vi "Main_v2.vi"() -> ()   [LabVIEW 2018]
uses:
  <vilib>/platform/TimedLoop/XDataNode/XDataNode.xnode
  <vilib>/Platform/TimedLoop/XDataNode/nitl_modes.ctl
  <vilib>/Platform/TimedLoop/XDataNode/XDNodeRunTimeDep.lvlib
  <vilib>/Platform/TimedLoop/XDataNode/wakeup.ctl
  <vilib>/Platform/TimedLoop/XDataNode/timing_clust.ctl
  Clusters/RoscoParams.ctl
  Clusters/SwapIn.ctl
  Clusters/SwapIndexes.ctl
  Clusters/FileDataChannel.ctl
  Clusters/SimulationConstants.ctl
panel:
  out "Generator Speed (rad/s)":sgl(slide)=7.06858e-05 scale=-4.0..4.0
  in  "?":T1(tab)
  out "Generator Speed":sgl(graph)
  out "Torque Setpoint (kNm)":sgl(graph)
  out "Pitch Setpoint":sgl(graph)
  in  "To VS_ControlMode":T2(ring)
  in  "Edit DISCON":bool
  out "DISCON.IN Contents":string
  in  "From VS_ControlMode":T2(ring)
  in  "GenSpeeed Amplitude":sgl=0.5
  in  "GenSpeed Mean":sgl=0.5
  out "Rotor Speed (rad/s)":sgl(slide)=7.06858e-05 scale=-4.0..4.0
  out "Torque Setpoint (kNm)":sgl(knob) scale=0.0..21586451.0
  out "Pitch Setpoint":sgl(knob) scale=0.0..1.5
  out "Power (kW)":sgl(slide) scale=-15000.0..15000.0 scale format="%.2f"
  in  "Init WindSpeed(m/s)":sgl=7.0
  in  "File path":path=path "/home/lvuser/rosco-tests"
  out "SimLoop Late?":bool
  out "FIFO Loop Late?":bool
  in  "Base filename":string="rosco-tests"
  out "Writing to cRIO?":bool
  in  "WriteData":bool
  in  "?":T3
  out "#RT FIFO":u32
  out "Call to Rosco Failed?":bool
  out "Rosco Return Message":string
  in  "?":bool
  out "time(s)":dbl
  out "RT Loop Late?":bool
  # "FOCAL Realtime Control (IEA 15MW)"
  # "SENSOR INPUTS"
  # "FILEWRITING SETTINGS"
  # "ERRORS"
  # "TURBINE SPECIFICATIONS"
  # "ROSCO OUTPUTS"
  # "RATED POWER: 15000000 W"
  # "RATED TORQUE: 19624046.66 Nm"
  # "RATED GEN SPEED: 0.79168 rad/s"
  # "ROSCO INPUTS"
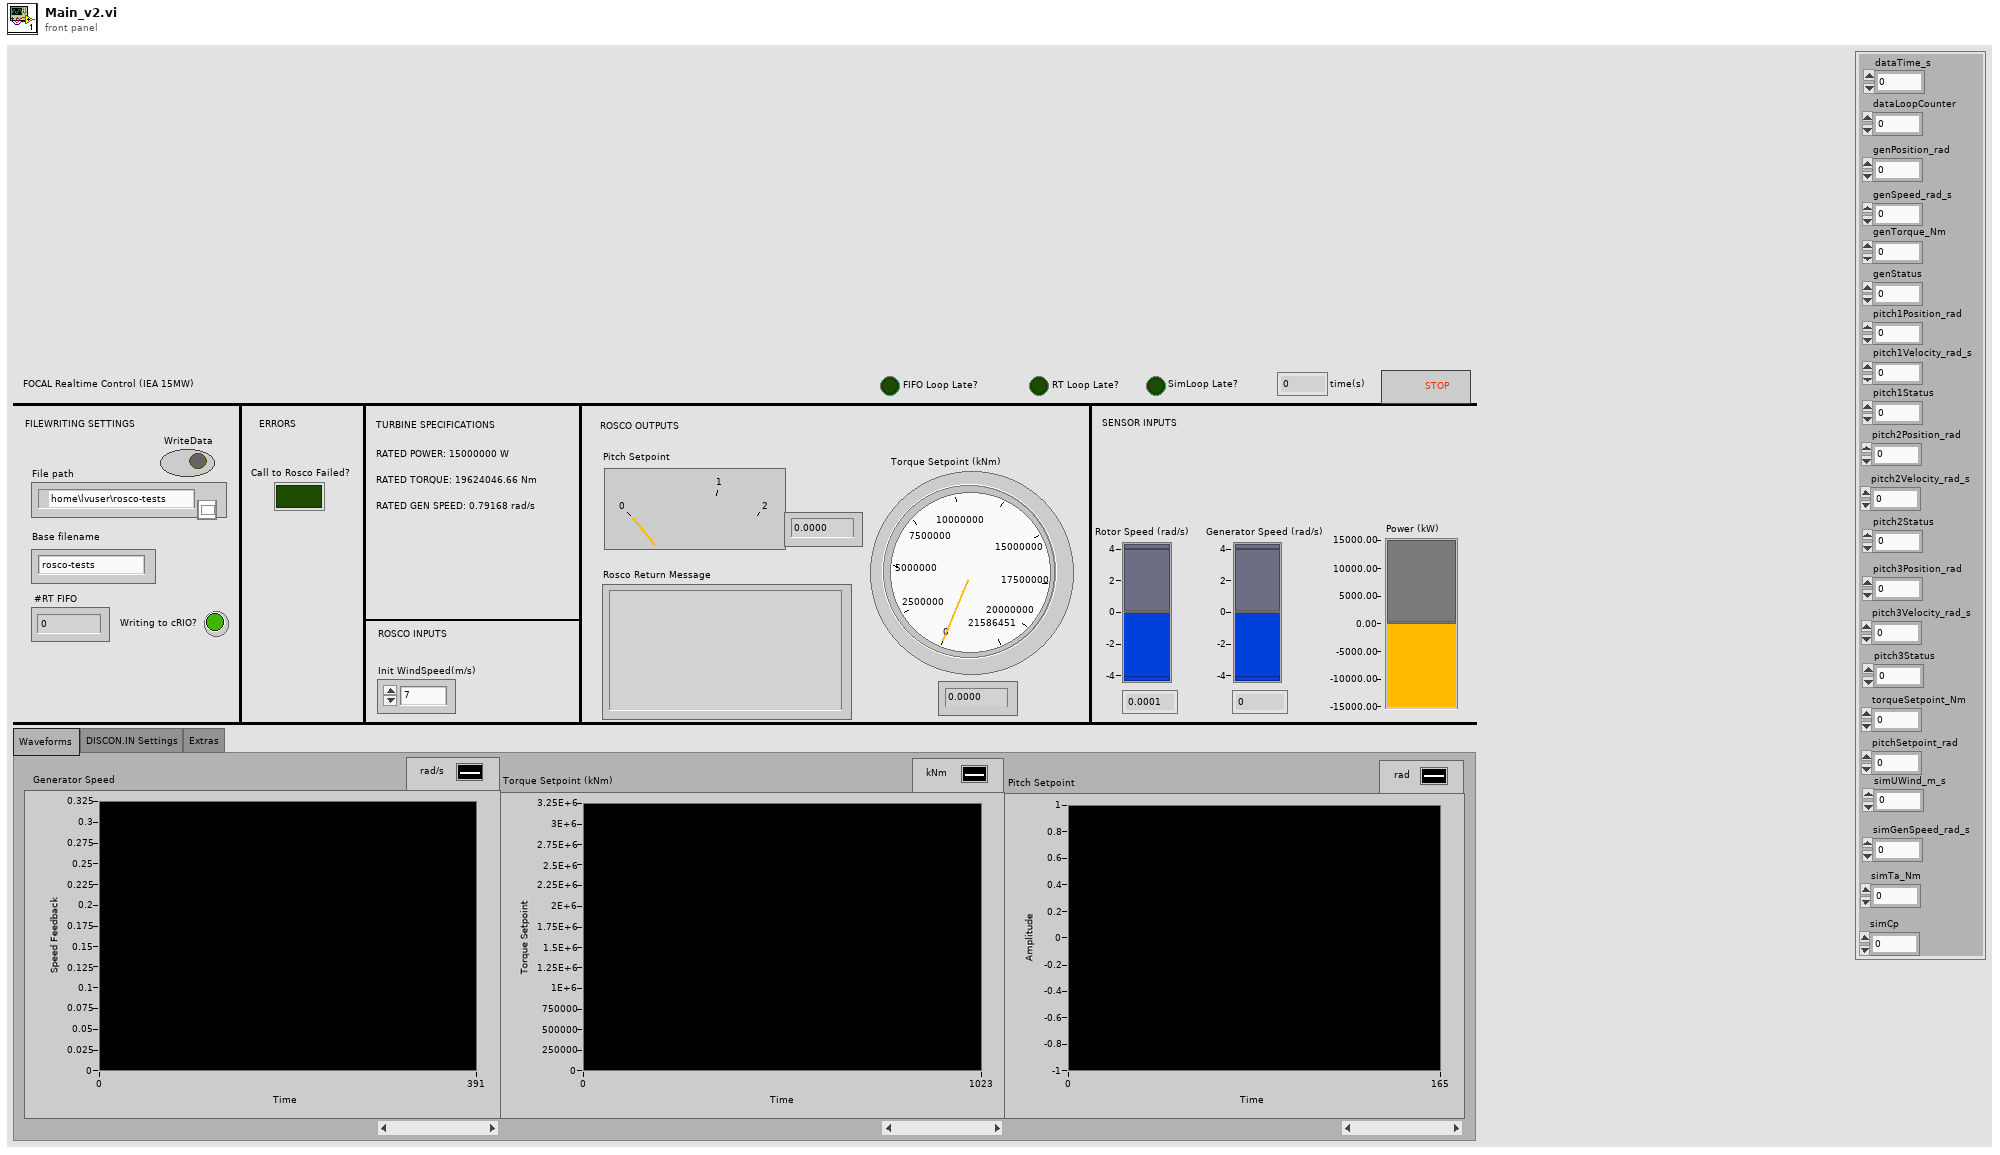
[diagram p1: front panel]
types:
  T1 = enum32{"Waveforms", "DISCON.IN Settings", "Extras"}
  T2 = enum16{"Constant Torque", "Constant Power", "PI Control"}
  T3 = typedef "FileDataChannel.ctl" = cluster{"genSpeed_rad_s":dbl, "genTorque_Nm":dbl, "dataLoopCounter":dbl, "genStatus":dbl, "pitch1Position_rad":dbl, "pitch1Velocity_rad_s":dbl, "pitch1Status":dbl, "dataTime_s":dbl, "genPosition_rad":dbl, "pitch2Position_rad":dbl, "pitch2Velocity_rad_s":dbl, "pitch2Status":dbl, "pitch3Position_rad":dbl, "pitch3Velocity_rad_s":dbl, "pitch3Status":dbl, "pitchSetpoint_rad":dbl, "torqueSetpoint_Nm":dbl, "simUWind_m_s":dbl, "simGenSpeed_rad_s":dbl, "simTa_Nm":dbl, "simCp":dbl}
  T4 = typedef "SwapIndexes.ctl" = cluster{"iSTATUS":i32, "TIME":i32, "DT":i32, "BL_PITCH_1":i32, "VS_MECHGENPWR":i32, "GEN_SPEED":i32, "ROT_SPEED":i32, "GENTQMEAS":i32, "Y_M":i32, "HORWINDV":i32, "ROOTMOOP1":i32, "ROOTMOOP2":i32, "BL_PITCH_2":i32, "BL_PITCH_3":i32, "ROOTMOOP3":i32, "INFILE_SIZE":i32, "FA_ACC":i32, "NUM_BLADES":i32, " OUT BL_PITCH":i32, "OUT_ TORQUE":i32, "OUTFILE_SIZE ":i32, "AVCMSG_SIZE":i32, "AERODYN TQ":i32, "VS_GENPWR":i32}
  T5 = typedef "SwapIn.ctl" = cluster{"BladePitch(rad)":sgl, "RotorSpeed(rad/s)":sgl, "GeneratorSpeed(rad/s)":sgl, " GeneratorTorque(Nm)":sgl, " Generator Power(W) ":sgl, " WindSpeed(m/s)":sgl, "aviMSGLength":sgl, "InfileLength":sgl, "OutfileLength":sgl, "iStatus":sgl, "Time":sgl, "Dt":sgl, "NumberofBlades":sgl}
  T6 = typedef "RoscoParams.ctl" = cluster{"avrSWAP":sgl[], "aviFAIL":i32, "avcMSG":string, "ReturnValue":i32}
  T7 = typedef "XDNodeRunTimeDep.lvlib/timing_clust.ctl" = cluster{"Expected End [f-1]":u64, "Actual End [f-1]":u64, "Finished Late? [f-1]":bool, "Expected End [i-1]":u64, "Actual End [i-1]":u64, "Finished Late? [i-1]":bool, "Expected Start [i]":u64, "Actual Start [i]":u64, "Expected Start [f]":u64, "Actual Start [f]":u64, "Source Name":string, "Structure Name":string, "Period":i64, "Deadline":i64, "Offset":i64, "Start":i64, "Priority":i32, "Timeout":i32, "Mode":T8, "Wakeup Reason":T9, "Error":errorcluster, "Source Type":string, "Secondary Source Type":string, "Global End Time":u64, "Global Start Time":u64, "Frame Duration":u64, "Iteration Duration":u64, "Assigned CPU":i32, "I/O Scan Engine Mode":u32}
  T8 = typedef "XDNodeRunTimeDep.lvlib/nitl_modes.ctl" = enum32{"No Change", "Process missed periods, maintain original phase", "Discard missed periods, maintain original phase", "Process missed periods, ignore original phase", "Discard missed periods, ignore original phase"}
  T9 = typedef "XDNodeRunTimeDep.lvlib/wakeup.ctl" = enum32{"Normal", "Aborted", "Asynchronous wakeup", "Timing source error", "Timed loop error", "Timeout"}
  T10 = typedef "SimulationConstants.ctl" = cluster{"Ngear":dbl, "RotorInertia":dbl, "GeneratorEff":dbl, "RotorRadius":sgl, "Rho":dbl, "NumBlades":i32, "ScaleFactor":dbl}
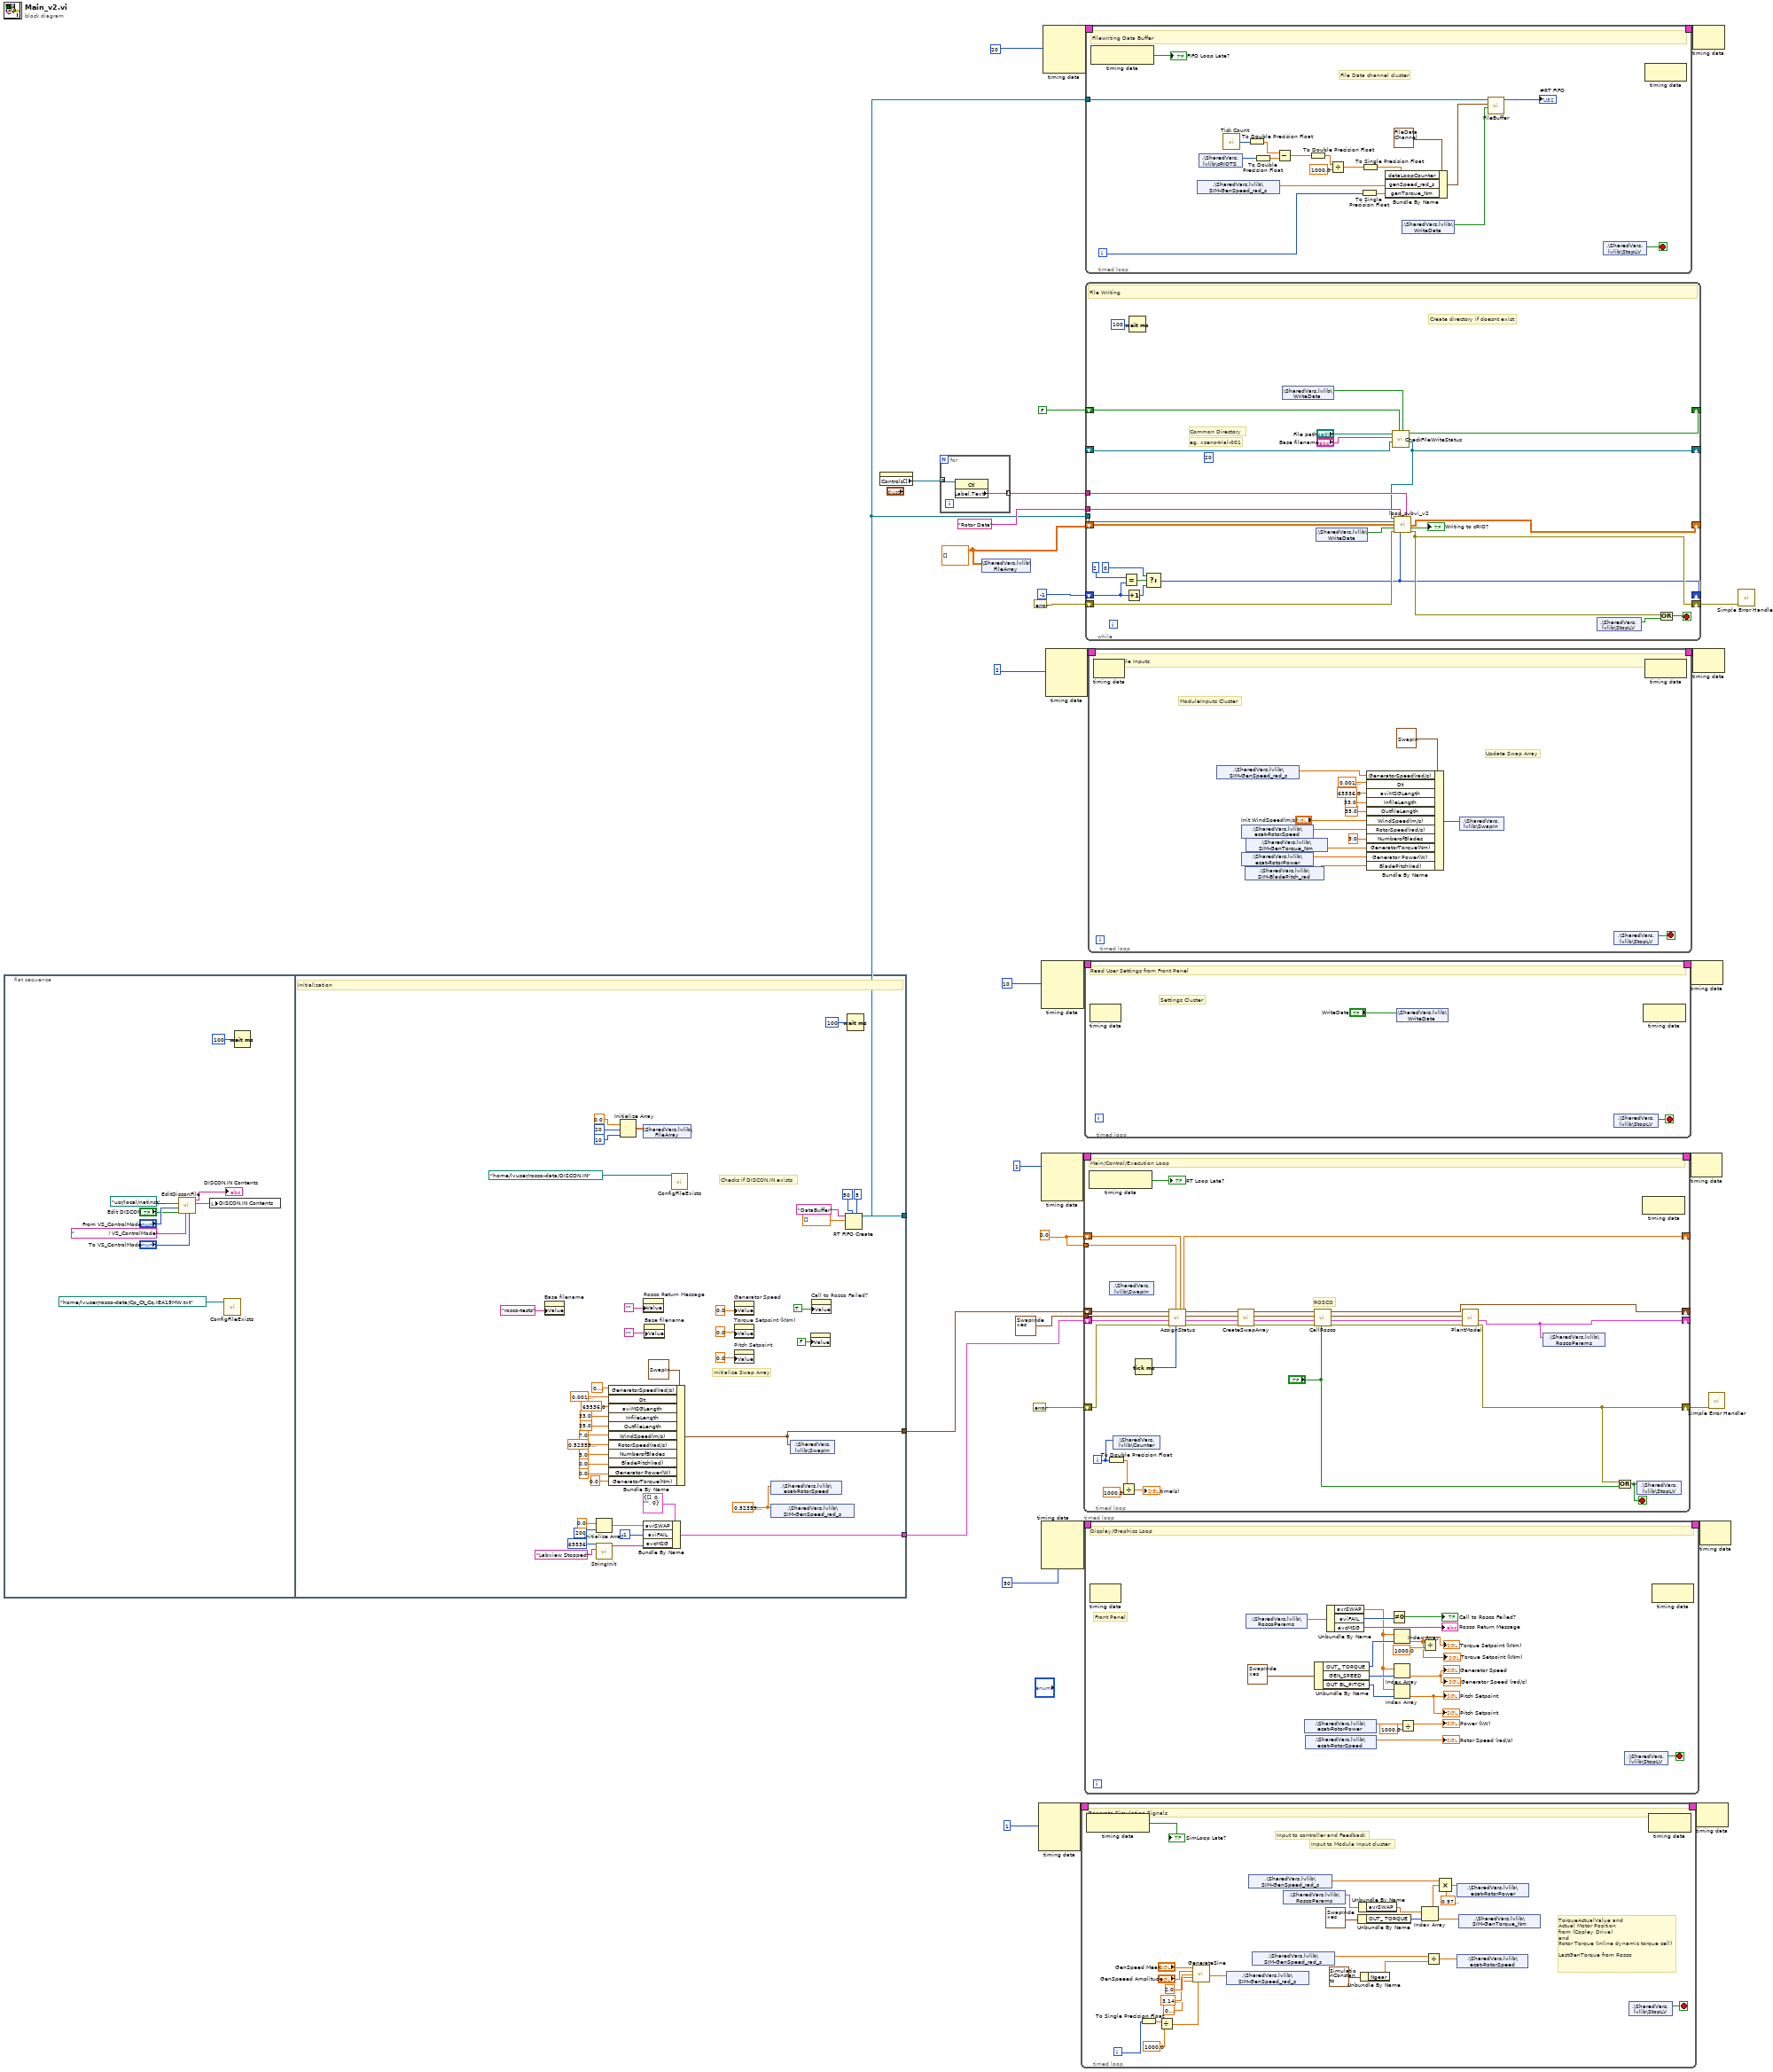
[diagram p0: block diagram]
diagram:
  w10 = dbl[][] [] ("File array 2")
  w17 = 0.0 ("y")
  (unwired) i64 20 ("Period")
  n1 = flat-sequence {
    tunnel: [w74] -> w11
    tunnel: [w47] -> w3
    tunnel: [w45] -> w2
    frame #0 {
      n2 = call "EditDisconFile.vi"("To VS_ControlMode"="To VS_ControlMode", "Append"="                   ! VS_ControlMode", "Edit DISCON"="Edit DISCON", "From VS_ControlMode"="From VS_ControlMode", "path"=path "/usr/local/natinst/labview/DISCON.IN") -> ("result string"=w36:string, "data"=→"DISCON.IN Contents":string)  [unwired: 4 in]
      n3 = local write "DISCON.IN Contents"(w36) -> ()
      n4 = call "ConfigFileExists.vi"("path"=path "/home/lvuser/rosco-data/Cp_Ct_Cq.IEA15MW.txt") -> ()  [unwired: 11 in]
      n5 = Wait (ms)(milliseconds to wait=u32 100) -> ()  [unwired: 1 out]
    }
    frame #1 {
      w43 = sgl 0.5236 ("RotorSpeed(rad/s)")
      # "Initialize Swap Array"
      # "Checks if DISCON.IN exists"
      # "Initialization"
      n6 = property on="Base filename" class="Str"("Value"="rosco-tests" ("Base filename")) -> ()  [unwired: 2 in, 2 out]
      n7 = Initialize Array(sgl 0.0 ("element"), 200 ("dimension size")) -> (w51:sgl[])
      n8 = call "StringInit.vi"("accOUTNAME"="Labview Stopped", "dimension size"=65536) -> ("result string"=w78:string)  [unwired: 9 in]
      n9 = Bundle By Name(cluster=T5 {"BladePitch(rad)"=0.0, "RotorSpeed(rad/s)"=0.0, "GeneratorSpeed(rad/s)"=0.0, " GeneratorTorque(Nm)"=0.0, " Generator Power(W) "=0.0, " WindSpeed(m/s)"=0.0, "aviMSGLength"=0.0, "InfileLength"=0.0, "OutfileLength"=0.0, "iStatus"=0.0, "Time"=0.0, "Dt"=0.0, "NumberofBlades"=0.0}, "GeneratorSpeed(rad/s)"=sgl 0.3, "Dt"=sgl 0.001, "aviMSGLength"=sgl 65536.0 ("new element/subarray"), "InfileLength"=sgl 33.0 ("new element/subarray"), "OutfileLength"=sgl 35.0 ("new element/subarray"), "WindSpeed(m/s)"=sgl 7.0, "RotorSpeed(rad/s)"=sgl 0.5236, "NumberofBlades"=sgl 3.0, "BladePitch(rad)"=sgl 0.0, "Generator Power(W)"=sgl 0.0, "GeneratorTorque(Nm)"=sgl 0.0) -> (w45:T5)
      n10 = Initialize Array(0.0 ("element"), 20 ("dimension size"), 10 ("dimension size")) -> (w70:dbl[][])
      n11 = shared-variable ".\\SharedVars.lvlib\\FileArray"(w70) -> ()  [unwired: 1 in, 1 out]
      n12 = Bundle By Name(cluster=T6 {"avrSWAP"=[], "aviFAIL"=0, "avcMSG"="", "ReturnValue"=0}, "avrSWAP"=w51, "aviFAIL"=-1, "avcMSG"=w78) -> (w47:T6)
      n13 = property on="Rosco Return Message" class="Str"("Value"="") -> ()  [unwired: 2 in, 2 out]
      n14 = property on="Base filename" class="Str"("Value"="") -> ()  [unwired: 2 in, 2 out]
      n15 = call "ConfigFileExists.vi"("path"=path "/home/lvuser/rosco-data/DISCON.IN") -> ()  [unwired: 11 in]
      n16 = property on="Generator Speed" class="WFChart (strict)"("Value"=sgl 0.0 ("Generator Speed")) -> ()  [unwired: 2 in, 2 out]
      n17 = property on="Torque Setpoint (kNm)" class="WFChart (strict)"("Value"=sgl 0.0 ("Generator Speed")) -> ()  [unwired: 2 in, 2 out]
      n18 = property on="Pitch Setpoint" class="WFChart (strict)"("Value"=sgl 0.0 ("Generator Speed")) -> ()  [unwired: 2 in, 2 out]
      n19 = shared-variable ".\\SharedVars.lvlib\\ecat-RotorSpeed"(w43) -> ()  [unwired: 1 in, 1 out]
      n20 = shared-variable ".\\SharedVars.lvlib\\SIM-GenSpeed_rad_s"(w43) -> ()  [unwired: 1 in, 1 out]
      n21 = shared-variable ".\\SharedVars.lvlib\\SwapIn"(w45) -> ()  [unwired: 1 in, 1 out]
      n22 = property class="Bool (strict)"("Value"=FALSE) -> ()  [unwired: 2 in, 2 out]
      n23 = property on="Call to Rosco Failed?" class="Bool (strict)"("Value"=TRUE ("Call to Rosco Failed?")) -> ()  [unwired: 2 in, 2 out]
      n24 = RT FIFO Create(0:"DataBuffer" ("name (unnamed)"), 1:dbl[] [] ("appended array"), 4:u32 50, 6:u32 5) -> (8:w74:refnum<k33>)  [unwired: 4 in, 2 out]
      n25 = Wait (ms)(milliseconds to wait=u32 100) -> ()  [unwired: 1 out]
    }
  }
  n26 = property class="Clust (strict)"() -> ("Controls[]"=w14:refnum<vi>[])  [unwired: 2 in, 2 out]
  n27 = for {
    tunnel: w14 -> [w86] mode=indexing
    tunnel: [w85] -> w13 mode=indexing
    n28 = property class="Ctl"(reference=w86) -> ("Label.Text"=w85:string)  [unwired: 1 in, 2 out]
  }
  n29 = shared-variable ".\\SharedVars.lvlib\\FileArray"(w10) -> ()  [unwired: 1 in, 1 out]
  n30 = node-c288(i64 1 ("Period")) -> (w25:T7)  [unwired: 3 in]
  n31 = node-c288(i64 1 ("Period")) -> (w23:T7)  [unwired: 3 in]
  n32 = node-c288(i64 10 ("Period")) -> (w29:T7)  [unwired: 3 in]
  n33 = node-c288(i64 50 ("Period")) -> (w27:T7)  [unwired: 3 in]
  n34 = node-c288(i64 20 ("Period")) -> (w33:T7)  [unwired: 3 in]
  n35 = node-c288(i64 2 ("Period")) -> (w31:T7)  [unwired: 3 in]
  n36 = timed-loop {
    timing: w25 -> [_]
    timing-out: [_] -> w24
    i -> [w108]
    stop <- w110 stop-if-true
    # "TorqueActualValue and \nActual Motor Position \nfrom (Copley Drive)\nand\nRotor Torque (Inline dynamic torque cell)\n\nLastGenTorque from Rosco"
    # "Input to Module Input cluster"
    # "Input to controller and Feedback"
    # "Generate Simulation Signals"
    n37 = node-c288() -> (→"SimLoop Late?":bool)  [unwired: 1 in]
    n38 = To Single Precision Float(number=w108) -> (single precision float=w109:sgl)
    n39 = Divide(x=w109, y=sgl 1000.0) -> (x/y=w102:sgl)
    n40 = call "GenerateSine.vi"("Mean"="GenSpeed Mean", "Amplitude"="GenSpeeed Amplitude", "frequency (f)"=sgl 2.0 ("value"), 9:sgl 3.14 ("value"), 11:sgl 0.1 ("value"), "time (s)"=w102) -> ("sine out"=w87:dbl)  [unwired: 9 in]
    n41 = shared-variable ".\\SharedVars.lvlib\\SIM-GenSpeed_rad_s"(w87) -> ()  [unwired: 1 in, 1 out]
    n42 = shared-variable ".\\SharedVars.lvlib\\SIM-GenSpeed_rad_s"() -> (w95:dbl)  [unwired: 1 in, 1 out]
    n43 = shared-variable ".\\SharedVars.lvlib\\SIM-GenSpeed_rad_s"() -> (w91:dbl)  [unwired: 1 in, 1 out]
    n44 = shared-variable ".\\SharedVars.lvlib\\RoscoParams"() -> (w94:T6)  [unwired: 1 in, 1 out]
    n45 = Unbundle By Name(T4 {"iSTATUS"=0, "TIME"=1, "DT"=2, "BL_PITCH_1"=3, "VS_MECHGENPWR"=13, "GEN_SPEED"=19, "ROT_SPEED"=20, "GENTQMEAS"=22, "Y_M"=23, "HORWINDV"=26, "ROOTMOOP1"=29, "ROOTMOOP2"=30, "BL_PITCH_2"=32, "BL_PITCH_3"=33, "ROOTMOOP3"=31, "INFILE_SIZE"=49, "FA_ACC"=52, "NUM_BLADES"=60, " OUT BL_PITCH"=44, "OUT_ TORQUE"=46, "OUTFILE_SIZE "=50, "AVCMSG_SIZE"=48, "AERODYN TQ"=89, "VS_GENPWR"=13} ("Index In")) -> ("OUT_ TORQUE"=w96:i32)
    n46 = Unbundle By Name(w94) -> ("avrSWAP"=w97:sgl[])
    n47 = Unbundle By Name(T10 {"Ngear"=1.0, "RotorInertia"=318628128.0, "GeneratorEff"=0.9700000286102295, "RotorRadius"=120.0, "Rho"=1.225000023841858, "NumBlades"=3, "ScaleFactor"=70.0} ("SimulationConst")) -> ("Ngear"=w89:dbl)
    n48 = Index Array(array=w97, index=w96) -> (element=w100:sgl)
    n49 = Divide(x=w91, y=w89) -> (x/y=w88:dbl)
    n50 = Compound Arithmetic op=MULTIPLY(w95, w100, sgl 0.97 ("value")) -> (w98:dbl)
    n51 = shared-variable ".\\SharedVars.lvlib\\ecat-RotorPower"(w98) -> ()  [unwired: 1 in, 1 out]
    n52 = shared-variable ".\\SharedVars.lvlib\\ecat-RotorSpeed"(w88) -> ()  [unwired: 1 in, 1 out]
    n53 = shared-variable ".\\SharedVars.lvlib\\SIM-GenTorque_Nm"(w100) -> ()  [unwired: 1 in, 1 out]
    n54 = shared-variable ".\\SharedVars.lvlib\\StopLV"() -> (w110:bool)  [unwired: 1 in, 1 out]
    n55 = node-c288() -> ()  [unwired: 1 in, 1 out]
  }
  n56 = timed-loop {
    timing: w23 -> [_]
    timing-out: [_] -> w22
    shift-right: [w128] -> _
    shift-left: w17 -> [w130]
    tunnel: w17 -> [w129]
    tunnel: T4 {"iSTATUS"=0, "TIME"=1, "DT"=2, "BL_PITCH_1"=3, "VS_MECHGENPWR"=13, "GEN_SPEED"=19, "ROT_SPEED"=20, "GENTQMEAS"=22, "Y_M"=23, "HORWINDV"=26, "ROOTMOOP1"=29, "ROOTMOOP2"=30, "BL_PITCH_2"=32, "BL_PITCH_3"=33, "ROOTMOOP3"=31, "INFILE_SIZE"=49, "FA_ACC"=52, "NUM_BLADES"=60, " OUT BL_PITCH"=44, "OUT_ TORQUE"=46, "OUTFILE_SIZE "=50, "AVCMSG_SIZE"=48, "AERODYN TQ"=89, "VS_GENPWR"=14} ("Index In") -> [w135]
    shift-right: [w115] -> _
    shift-left: w3 -> [w134]
    shift-right: [w119] -> _
    shift-left: w2 -> [w114]
    shift-right: [w118] -> w4
    shift-left: errorcluster {"status"=FALSE, "code"=0, "source"=""} ("error out") -> [w125]
    i -> [w117]
    stop <- w123 stop-if-true
    # "ROSCO"
    # "Main/Control/Execution Loop"
    n57 = node-c288() -> (→"RT Loop Late?":bool)  [unwired: 1 in]
    n58 = To Double Precision Float(number=w117) -> (double precision float=w141:dbl)
    n59 = shared-variable ".\\SharedVars.lvlib\\SwapIn"() -> ()  [unwired: 1 in, 2 out]
    n60 = shared-variable ".\\SharedVars.lvlib\\Counter"(w117) -> ()  [unwired: 1 in, 1 out]
    n61 = Divide(x=w141, y=1000.0) -> (x/y=→"time(s)":dbl)
    n62 = Tick Count (ms)() -> (millisecond timer value=w116:u32)
    n63 = call "AssignStatus.vi"("LoopCount"=w130, "Time"=w116, "Init Val"=w129, "error in (no error)"=w125, "ROSCO Params"=w134, 10:w135, "SwapIn"=w114) -> ("error out"=w138:errorcluster, "ROSCO Params 2"=w132:T6, 2:w133:T4, "SwapIn"=w137:T5, "Count+1"=w128:dbl)
    n64 = call "CreateSwapArray.vi"("error in (no error)"=w138, "ROSCO Params"=w132, "Index In"=w133, "SwapIn"=w137) -> ("error out"=w131:errorcluster, "ROSCO Params Out"=w136:T6, "Index Out"=w126:T4, "SwapIn Out"=w127:T5)  [unwired: 4 in]
    n65 = call "CallRosco.vi"("StopLV"="?", "error in (no error)"=w131, "ROSCO Params in"=w136, "Index In"=w126, "SwapIn"=w127) -> ("error out"=w122:errorcluster, "ROSCO Params out"=w121:T6, "IndexOut"=w120:T4, "SwapOut"=w119:T5)  [unwired: 3 in]
    n66 = call "PlantModel.vi"("error in (no error)"=w122, "ROSCO Params in"=w121, 9:w120) -> ("error out"=w118:errorcluster, "ROSCO Params out"=w115:T6)  [unwired: 5 in, 1 out]
    n67 = shared-variable ".\\SharedVars.lvlib\\RoscoParams"(w115) -> ()  [unwired: 1 in, 1 out]
    n68 = Or(x=w118, y="?") -> (x .or. y?=w123:bool)
    n69 = shared-variable ".\\SharedVars.lvlib\\StopLV"(w123) -> ()  [unwired: 1 in, 1 out]
    n70 = node-c288() -> ()  [unwired: 1 in, 1 out]
  }
  n71 = timed-loop {
    timing: w29 -> [_]
    timing-out: [_] -> w28
    stop <- w147 stop-if-true
    # "Settings Cluster"
    # "Read User Settings from Front Panel"
    n72 = node-c288() -> ()  [unwired: 1 in, 1 out]
    n73 = shared-variable ".\\SharedVars.lvlib\\WriteData"("WriteData") -> ()  [unwired: 1 in, 1 out]
    n74 = shared-variable ".\\SharedVars.lvlib\\StopLV"() -> (w147:bool)  [unwired: 1 in, 1 out]
    n75 = node-c288() -> ()  [unwired: 1 in, 1 out]
  }
  n76 = timed-loop {
    timing: w27 -> [_]
    timing-out: [_] -> w26
    stop <- w167 stop-if-true
    # "Front Panel"
    # "Display/Graphics Loop"
    n77 = node-c288() -> ()  [unwired: 1 in, 1 out]
    n78 = shared-variable ".\\SharedVars.lvlib\\RoscoParams"() -> (w166:T6)  [unwired: 1 in, 1 out]
    n79 = shared-variable ".\\SharedVars.lvlib\\ecat-RotorPower"() -> (w157:sgl)  [unwired: 1 in, 1 out]
    n80 = shared-variable ".\\SharedVars.lvlib\\ecat-RotorSpeed"() -> (→"Rotor Speed (rad/s)":sgl)  [unwired: 1 in, 1 out]
    n81 = Unbundle By Name(T4 {"iSTATUS"=0, "TIME"=1, "DT"=2, "BL_PITCH_1"=3, "VS_MECHGENPWR"=13, "GEN_SPEED"=19, "ROT_SPEED"=20, "GENTQMEAS"=22, "Y_M"=23, "HORWINDV"=26, "ROOTMOOP1"=29, "ROOTMOOP2"=30, "BL_PITCH_2"=32, "BL_PITCH_3"=33, "ROOTMOOP3"=31, "INFILE_SIZE"=49, "FA_ACC"=52, "NUM_BLADES"=60, " OUT BL_PITCH"=44, "OUT_ TORQUE"=46, "OUTFILE_SIZE "=50, "AVCMSG_SIZE"=48, "AERODYN TQ"=89, "VS_GENPWR"=14} ("Index In")) -> ("OUT_ TORQUE"=w165:i32, "GEN_SPEED"=w164:i32, "OUT BL_PITCH"=w159:i32)
    n82 = Unbundle By Name(w166) -> ("avrSWAP"=w160:sgl[], "aviFAIL"=w162:i32, "avcMSG"=→"Rosco Return Message":string)
    n83 = Not Equal To 0?(x=w162) -> (x != 0?=→"Call to Rosco Failed?":bool)
    n84 = Index Array(array=w160, index=w165) -> (element=w151:sgl)
    "Torque Setpoint (kNm)" <- w151
    "Torque Setpoint (kNm)" <- w151
    n85 = Index Array(array=w160, index=w164) -> (element=→"Generator Speed" →"Generator Speed (rad/s)":sgl)
    n86 = Index Array(array=w160, index=w159) -> (element=→"Pitch Setpoint" →"Pitch Setpoint":sgl)
    n87 = Divide(x=w157, y=sgl 1000.0) -> (x/y=→"Power (kW)":sgl)
    n88 = Divide(x=w151, y=sgl 1000.0) -> ()  [unwired: 1 out]
    n89 = shared-variable ".\\SharedVars.lvlib\\StopLV"() -> (w167:bool)  [unwired: 1 in, 1 out]
    n90 = node-c288() -> ()  [unwired: 1 in, 1 out]
  }
  n91 = while {
    shift-right: [w170] -> _
    shift-left: _ -> [w171]
    shift-right: [w178] -> _
    shift-left: FALSE -> [w179]
    shift-right: [w191] -> w6
    shift-left: errorcluster {"status"=FALSE, "code"=0, "source"=""} ("error out") -> [w190]
    tunnel: "Rotor Data" -> [w173]
    tunnel: w13 -> [w174]
    tunnel: w11 -> [w175]
    shift-right: [w187] -> _
    shift-left: -1 -> [w189]
    shift-right: [w182] -> _
    shift-left: w10 -> [w188]
    stop <- w193 stop-if-true
    # "eg. xsens-trial-001"
    # "Create directory if doesnt exist"
    # "Common Directory"
    # "File Writing"
    n92 = Equal?(x=2 ("t"), y=w189) -> (x = y?=w184:bool)
    n93 = Increment(x=w189) -> (x+1=w183:i32)
    n94 = Wait (ms)(milliseconds to wait=u32 100) -> ()  [unwired: 1 out]
    n95 = Select(t=0, s=w184, f=w183) -> (s? t:f=w187:i32)
    n96 = shared-variable ".\\SharedVars.lvlib\\WriteData"() -> (w180:bool)  [unwired: 1 in, 1 out]
    n97 = shared-variable ".\\SharedVars.lvlib\\WriteData"() -> (w176:bool)  [unwired: 1 in, 1 out]
    n98 = call "CheckFIleWriteStatus.vi"("WriteDataButtonVal"=w180, "WritePrevVal"=w179, "Refnum in"=w171, "Base filename"="Base filename", "File path"="File path") -> ("Refnum out"=w170:refnum<k34>, "WriteCurrentVal"=w178:bool)  [unwired: 4 in, 1 out]
    n99 = call "loop_subvi_v2.vi"("Refnum in"=w170, "Group Name"=w173, "Channel Names"=w174, "rt fifo"=w175, "File array"=w188, "Write?"=w176, "error in (no error)"=w190, "index"=w187) -> ("File array 2"=w182:dbl[][], "Writing to file"=→"Writing to cRIO?":bool, "error out"=w191:errorcluster)  [unwired: 4 in, 1 out]
    n100 = shared-variable ".\\SharedVars.lvlib\\StopLV"() -> (w194:bool)  [unwired: 1 in, 1 out]
    n101 = Or(x=w191, y=w194) -> (x .or. y?=w193:bool)
  }
  n102 = timed-loop {
    timing: w33 -> [_]
    timing-out: [_] -> w32
    tunnel: w11 -> [w201]
    i -> [w196]
    stop <- w213 stop-if-true
    # "File Data channel cluster"
    # "Filewriting Data Buffer"
    n103 = node-c288() -> (→"FIFO Loop Late?":bool)  [unwired: 1 in]
    n104 = shared-variable ".\\SharedVars.lvlib\\SIM-GenSpeed_rad_s"() -> (w206:dbl)  [unwired: 1 in, 1 out]
    n105 = shared-variable ".\\SharedVars.lvlib\\cRIOTS"() -> (w208:u64)  [unwired: 1 in, 1 out]
    n106 = call "Tick Count"() -> ("Tick Count(mSec)"=w209:u32)
    n107 = To Double Precision Float(number=w209) -> (double precision float=w198:dbl)
    n108 = To Double Precision Float(number=w208) -> (double precision float=w207:dbl)
    n109 = Subtract(x=w198, y=w207) -> (x-y=w210:dbl)
    n110 = To Double Precision Float(number=w210) -> (double precision float=w212:dbl)
    n111 = Divide(x=w212, y=1000.0) -> (x/y=w197:dbl)
    n112 = To Single Precision Float(number=w196) -> (single precision float=w199:sgl)
    n113 = To Single Precision Float(number=w197) -> (single precision float=w205:sgl)
    n114 = Bundle By Name(cluster=T3 {"genSpeed_rad_s"=0.0, "genTorque_Nm"=0.0, "dataLoopCounter"=0.0, "genStatus"=0.0, "pitch1Position_rad"=0.0, "pitch1Velocity_rad_s"=0.0, "pitch1Status"=0.0, "dataTime_s"=0.0, "genPosition_rad"=0.0, "pitch2Position_rad"=0.0, "pitch2Velocity_rad_s"=0.0, "pitch2Status"=0.0, "pitch3Position_rad"=0.0, "pitch3Velocity_rad_s"=0.0, "pitch3Status"=0.0, "pitchSetpoint_rad"=0.0, "torqueSetpoint_Nm"=0.0, "simUWind_m_s"=0.0, "simGenSpeed_rad_s"=0.0, "simTa_Nm"=0.0, "simCp"=0.0} ("SwapIn"), "dataLoopCounter"=w205, "genSpeed_rad_s"=w206, "genTorque_Nm"=w199) -> (w203:T3)
    n115 = shared-variable ".\\SharedVars.lvlib\\WriteData"() -> (w202:bool)  [unwired: 1 in, 1 out]
    n116 = call "FileBuffer.vi"("Boolean"=w202, "FileDataChannel"=w203, "Refnum in"=w201) -> ("# elements"=→"#RT FIFO":u32)  [unwired: 7 in, 1 out]
    n117 = shared-variable ".\\SharedVars.lvlib\\StopLV"() -> (w213:bool)  [unwired: 1 in, 1 out]
    n118 = node-c288() -> ()  [unwired: 1 in, 1 out]
  }
  n119 = timed-loop {
    timing: w31 -> [_]
    timing-out: [_] -> w30
    stop <- w230 stop-if-true
    # "Update Swap Array"
    # "ModuleInputs Cluster"
    # "Read Module Inputs"
    n120 = node-c288() -> ()  [unwired: 1 in, 1 out]
    n121 = shared-variable ".\\SharedVars.lvlib\\SIM-GenSpeed_rad_s"() -> (w222:dbl)  [unwired: 1 in, 1 out]
    n122 = shared-variable ".\\SharedVars.lvlib\\ecat-RotorSpeed"() -> (w217:sgl)  [unwired: 1 in, 1 out]
    n123 = shared-variable ".\\SharedVars.lvlib\\ecat-RotorPower"() -> (w219:sgl)  [unwired: 1 in, 1 out]
    n124 = shared-variable ".\\SharedVars.lvlib\\SIM-BladePitch_rad"() -> (w218:dbl)  [unwired: 1 in, 1 out]
    n125 = shared-variable ".\\SharedVars.lvlib\\SIM-GenTorque_Nm"() -> (w220:dbl)  [unwired: 1 in, 1 out]
    n126 = Bundle By Name(cluster=T5 {"BladePitch(rad)"=0.0, "RotorSpeed(rad/s)"=0.0, "GeneratorSpeed(rad/s)"=0.0, " GeneratorTorque(Nm)"=0.0, " Generator Power(W) "=0.0, " WindSpeed(m/s)"=0.0, "aviMSGLength"=0.0, "InfileLength"=0.0, "OutfileLength"=0.0, "iStatus"=0.0, "Time"=0.0, "Dt"=0.0, "NumberofBlades"=0.0}, "GeneratorSpeed(rad/s)"=w222, "Dt"=sgl 0.001, "aviMSGLength"=sgl 65536.0 ("new element/subarray"), "InfileLength"=sgl 33.0 ("new element/subarray"), "OutfileLength"=sgl 35.0 ("new element/subarray"), "WindSpeed(m/s)"="Init WindSpeed(m/s)", "RotorSpeed(rad/s)"=w217, "NumberofBlades"=sgl 3.0, "GeneratorTorque(Nm)"=w220, "Generator Power(W)"=w219, "BladePitch(rad)"=w218) -> (w229:T5)
    n127 = shared-variable ".\\SharedVars.lvlib\\SwapIn"(w229) -> ()  [unwired: 1 in, 1 out]
    n128 = shared-variable ".\\SharedVars.lvlib\\StopLV"() -> (w230:bool)  [unwired: 1 in, 1 out]
    n129 = node-c288() -> ()  [unwired: 1 in, 1 out]
  }
  n130 = node-c288(w22) -> ()  [unwired: 1 out]
  n131 = node-c288(w28) -> ()  [unwired: 1 out]
  n132 = node-c288(w32) -> ()  [unwired: 1 out]
  n133 = node-c288(w30) -> ()  [unwired: 1 out]
  n134 = node-c288(w24) -> ()  [unwired: 1 out]
  n135 = node-c288(w26) -> ()  [unwired: 1 out]
  n136 = call <vilib>:"Simple Error Handler.vi"("error in (no error)"=w4) -> ()  [unwired: 4 in, 5 out]
  n137 = call <vilib>:"Simple Error Handler.vi"("error in (no error)"=w6) -> ()  [unwired: 4 in, 5 out]
